vi "simx Get Out Message Info.vi"(8 "error in (no error)":errorcluster, 9 "info":i32, 10 "infoType":i32, 11 "clientID":i32) -> (0 "error out":errorcluster, 1 "info out":i32, 3 "function return":i32)   [LabVIEW 2019, in "PXL_V-REP.lvlib"]
doc: "EXTAPI_DLLEXPORT simxInt simxGetOutMessageInfo(simxInt clientID,simxInt infoType,simxInt* info);"
uses:
  PXL_V-REP.lvlib
  <userlib>/V-REP/remoteApi.dll
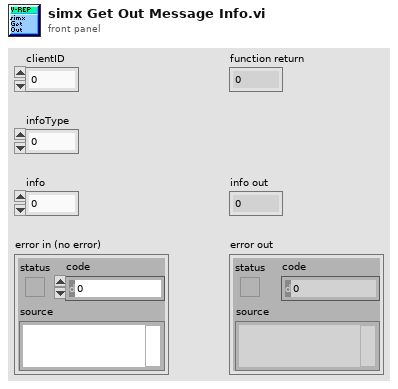
[diagram p1: front panel]
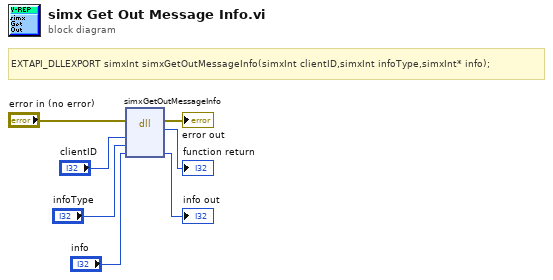
[diagram p0: block diagram]
diagram:
  # "EXTAPI_DLLEXPORT simxInt simxGetOutMessageInfo(simxInt clientID,simxInt infoType,simxInt* info);"
  n1 = dll-call lib="C:/Program Files (x86)/National Instruments/LabVIEW 2019/user.lib/V-REP/remoteApi.*" fn="simxGetOutMessageInfo"(error in="error in (no error)", "clientID"="clientID", "infoType"="infoType", "info"="info") -> (error out=→"error out":errorcluster, →"function return":i32, "info"=→"info out":i32)  [unwired: 4 in, 1 out]
